vi "Initalize.vi"(8 "error in (no error)":errorcluster, 9 "Section":string, 10 "Config Path":path, 11 "Motion Controller in":refnum<class "Parent SIM Motion Controller.lvclass">) -> (0 "error out":errorcluster, 3 "Motion Controller out":refnum<class "Parent SIM Motion Controller.lvclass">)   [LabVIEW 2022 SP3, in "Parent SIM Motion Controller.lvclass"]
uses:
  Parent SIM Motion Controller.lvclass
  C:/Stage-Work/MAS/Base/Base.lvclass
  Axis Data.ctl
  Axis Parameters.ctl
  Axis Settings.ctl
  Base/Base.lvclass/Base.ctl
  Parent SIM Motion Controller.lvclass/Parent SIM Motion Controller.ctl
  Base/Accessors/Write Config Path.vi
  Base/Accessors/Write Section.vi
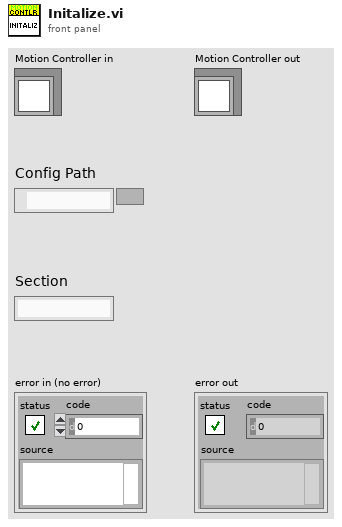
[diagram p1: front panel]
types:
  T1 = typedef "Parent SIM Motion Controller.lvclass/Axis Data.ctl" = cluster{"Axis Parameters":T2, "Axis Settings":T3, "Time Stamp":timestamp}
  T2 = typedef "Parent SIM Motion Controller.lvclass/Axis Parameters.ctl" = cluster{"Moving":bool, "Homed":bool, "Desired Position":dbl, "Current Positon":dbl, "Current Speed":dbl}
  T3 = typedef "Parent SIM Motion Controller.lvclass/Axis Settings.ctl" = cluster{"Speed":dbl, "Acceleration":dbl}
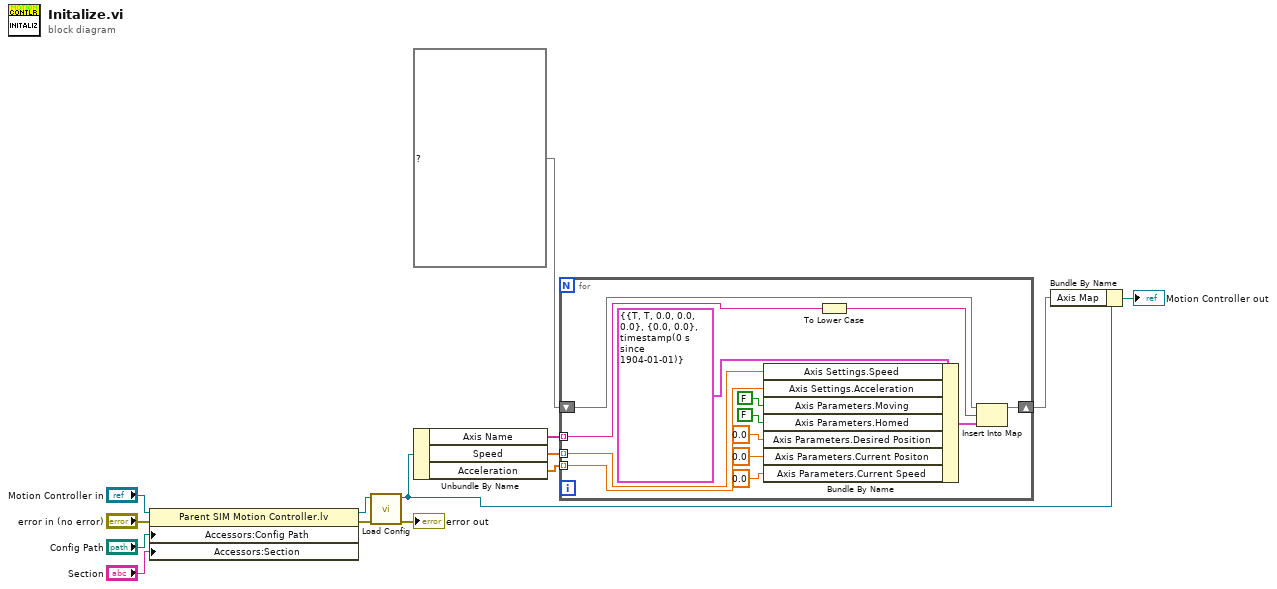
[diagram p0: block diagram]
diagram:
  n1 = property class="Parent SIM Motion Controller.lv"(reference="Motion Controller in", error in="error in (no error)", "Accessors:Config Path"="Config Path", "Accessors:Section"="Section") -> (reference out=w10:refnum<class "Parent SIM Motion Controller.lvclass">, error out=w12:errorcluster)
  n2 = call-dynamic "Load Config.vi"("error in (no error)"=w12, "Motion Controller in"=w10) -> ("error out"=→"error out":errorcluster, "Motion Controller out"=w7:refnum<class "Parent SIM Motion Controller.lvclass">)  [unwired: 8 in]
  n3 = Unbundle By Name(w7) -> ("Axis Name"=w6:string[], "Speed"=w5:dbl[], "Acceleration"=w4:dbl[])
  n4 = for {
    tunnel: w6 -> [w25] mode=indexing
    tunnel: w5 -> [w27] mode=indexing
    tunnel: w4 -> [w26] mode=indexing
    shift-right: [w22] -> w1
    shift-left: map{string, T1} {} ("map") -> [w23]
    n5 = Bundle By Name(cluster=T1 {"Axis Parameters"={"Moving"=TRUE, "Homed"=TRUE, "Desired Position"=0.0, "Current Positon"=0.0, "Current Speed"=0.0}, "Axis Settings"={"Speed"=0.0, "Acceleration"=0.0}, "Time Stamp"=timestamp(0 s since 1904-01-01)} ("Axis Data"), "Axis Settings.Speed"=w27, "Axis Settings.Acceleration"=w26, "Axis Parameters.Moving"=FALSE, "Axis Parameters.Homed"=FALSE, "Axis Parameters.Desired Position"=0.0, "Axis Parameters.Current Positon"=0.0, "Axis Parameters.Current Speed"=0.0) -> (w15:T1)
    n6 = To Lower Case(string=w25) -> (all lower case string=w24:string)
    n7 = Insert Into Map(map in=w23, key=w24, value=w15) -> (map out=w22:map{string, T1})  [unwired: 2 out]
  }
  n8 = Bundle By Name(cluster=w7, "Axis Map"=w1) -> (→"Motion Controller out":refnum<class "Parent SIM Motion Controller.lvclass">)
